vi "Microsync send packet.vi"(7 "Command":string="GET", 8 "error in (no error)":errorcluster, 10 "Arguments":T1, 11 "VISA resource name":refnum<visa-resource-name>) -> (0 "error out":errorcluster, 2 "return count":u32, 3 "VISA resource name out":refnum<visa-resource-name>)   [LabVIEW 2023]
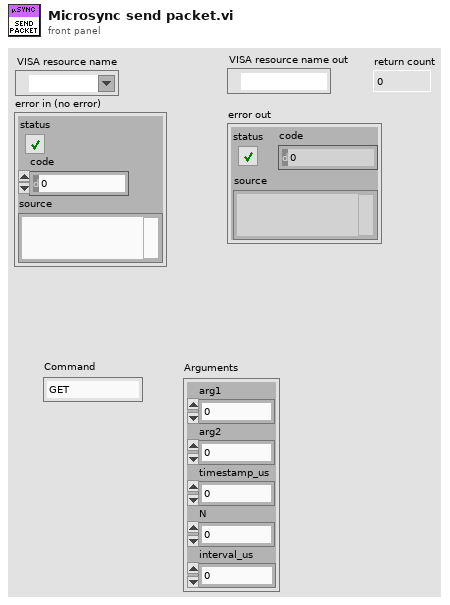
[diagram p1: front panel]
types:
  T1 = cluster{"interval_us":u32, "N":u32, "timestamp_us":u32, "arg2":u32, "arg1":u32}
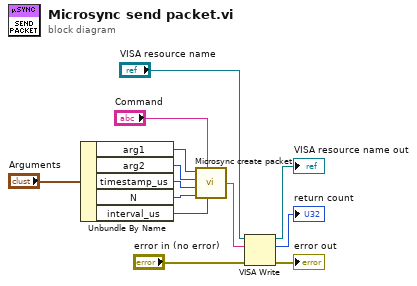
[diagram p0: block diagram]
diagram:
  n1 = Unbundle By Name("Arguments") -> ("arg1"=w6:u32, "arg2"=w5:u32, "timestamp_us"=w4:u32, "N"=w3:u32, "interval_us"=w2:u32)
  n2 = call "Microsync create packet.vi"("interval_us"=w2, "Command"="Command", "N"=w3, "timestamp_us"=w4, "arg2"=w5, "arg1"=w6) -> ("data packet"=w13:string)
  n3 = VISA Write(VISA resource name="VISA resource name", write buffer=w13, error in (no error)="error in (no error)") -> (VISA resource name out=→"VISA resource name out":refnum<visa-resource-name>, return count=→"return count":u32, error out=→"error out":errorcluster)
